vi "GetStepResults.vi"(11 "Sequence Context In":refnum<k7>) -> (0 "error out":errorcluster, 2 "String Value Step Result":string, 3 "Numeric Limit Step Result":dbl format="%.2f")   [LabVIEW 2011]
doc: "This VI demonstrates how to cast a SequenceFile object in order access properties of the PropertyObjectFile and PropertyObject parent classes"
uses:
  <vilib>/addons/TestStand/_TSUtility.llb/TestStand - Get Property Value (Number).vi
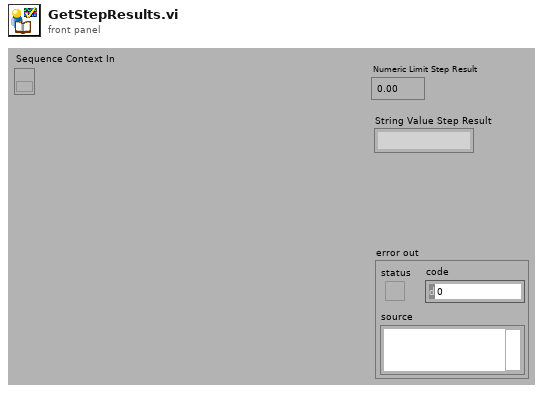
[diagram p1: front panel]
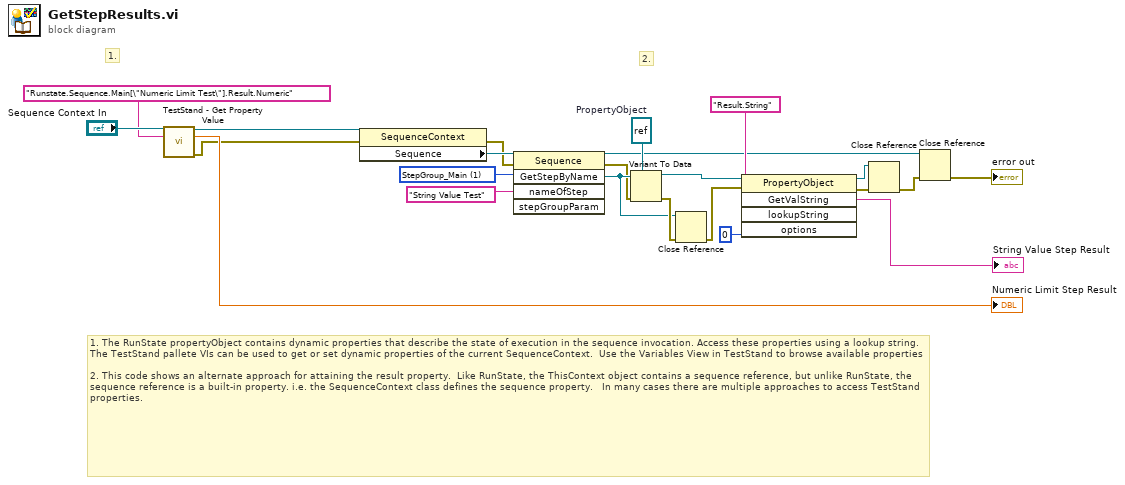
[diagram p0: block diagram]
diagram:
  w10 = 1 items=["StepGroup_Setup", "StepGroup_Main", "StepGroup_Cleanup"] ("stepGroupParam")
  w18 = refnum<k7> refnum  # PropertyObject
  # "2."
  # "1."
  # "1. The RunState propertyObject contains dynamic properties that describe the state of execution in the sequence invocation. Access these properties using a lookup string.  The TestStand pallete VIs can be used to get or set dynamic properties of the current SequenceContext.  Use the Variables View in TestStand to browse available properties\n\n2. This code shows an alternate approach for attaining the result property.  Like RunState, the ThisContext object contains a sequence reference, but unlike RunState, the sequence reference is a built-in property. i.e. the SequenceContext class defines the sequence property.   In many cases there are multiple approaches to access TestStand properties."
  n1 = call-poly <vilib>:"TestStand - Get Property Value.vi"("Sequence Context In"="Sequence Context In", "Lookup String"="Runstate.Sequence.Main[\"Numeric Limit Test\"].Result.Numeric") -> ("Sequence Context Out"=w21:refnum<k7>, "Value"=→"Numeric Limit Step Result":dbl, "error out"=w9:errorcluster)  [unwired: 11 in]
  n2 = property class="SequenceContext"(reference=w21, error in=w9) -> (error out=w8:errorcluster, "Sequence"=w20:refnum<k7>)  [unwired: 1 out]
  n3 = invoke class="Sequence" method="GetStepByName"(reference=w20, error in=w8, "nameOfStep"="String Value Test", "stepGroupParam"=w10) -> (reference out=w5:refnum<k7>, error out=w1:errorcluster, "GetStepByName"=w16:refnum<k7>)  [unwired: 1 in, 2 out]
  n4 = Variant To Data(error in=w1, type=w18, Variant=w16) -> (data=w15:refnum<k7>, error out=w17:errorcluster)
  n5 = Close Reference(reference=w16, error in (no error)=w17) -> (error out=w14:errorcluster)
  n6 = invoke class="PropertyObject" method="GetValString"(reference=w15, error in=w14, "lookupString"="Result.String" ("Lookup String"), "options"=0) -> (reference out=w7:refnum<k7>, error out=w6:errorcluster, "GetValString"=→"String Value Step Result":string)  [unwired: 1 in, 2 out]
  n7 = Close Reference(reference=w7, error in (no error)=w6) -> (error out=w4:errorcluster)
  n8 = Close Reference(reference=w5, error in (no error)=w4) -> (error out=→"error out":errorcluster)
